vi "is_inside.vi"(8 "error in (no error)":errorcluster, 10 "SpaceVector.lvclass":refnum<class "SpaceVector.lvclass">, 11 "ROI in":refnum<class "RoiEllipsoid.lvclass">=refnum) -> (0 "error out":errorcluster, 2 "is inside?":bool, 3 "ROI out":refnum<class "RoiEllipsoid.lvclass">)   [LabVIEW 2010, in "RoiEllipsoid.lvclass"]
uses:
  RoiEllipsoid.lvclass
  common/classes/SpaceVector/SpaceVector/SpaceVector.lvclass
  RoiGeneric/RoiGeneric.lvclass
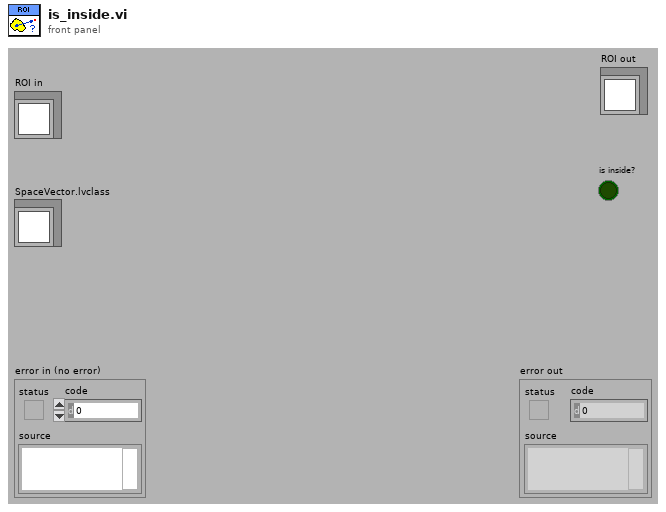
[diagram p1: front panel]
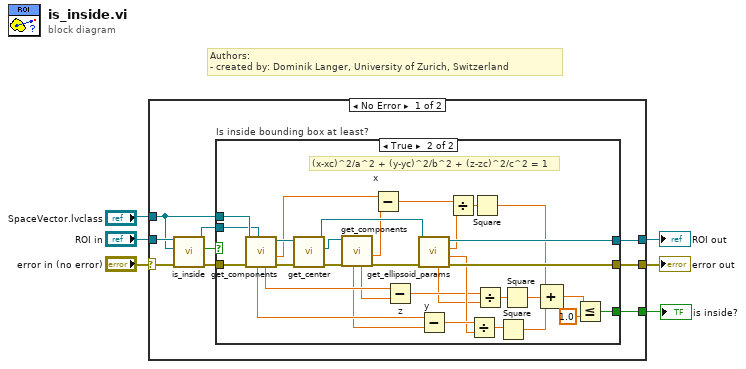
[diagram p0: block diagram]
diagram:
  # "Authors: \n- created by: Dominik Langer, University of Zurich, Switzerland"
  n1 = case shown="No Error" "error in (no error)" {
    selector: "error in (no error)" -> [w15 w50]
    tunnel: "ROI in" -> [w14 w49]
    tunnel: "SpaceVector.lvclass" -> [w13 _]
    tunnel: [w10 w50] -> w3
    tunnel: [w8 w49] -> w2
    tunnel: [w7 _] -> w1
    frame No Error {
      n2 = call-parent "is_inside.vi"("error in (no error)"=w15, "SpaceVector.lvclass"=w13, "ROI in"=w14) -> ("error out"=w12:errorcluster, "is inside?"=w11:bool, "ROI out"=w9:refnum<class "RoiEllipsoid.lvclass">)  [unwired: 6 in]
      n3 = case "Is inside bounding box at least?" shown="True" w11 {
        tunnel: w13 -> [_ w48]
        tunnel: w12 -> [w17 w47]
        tunnel: [w17 w46] -> w10
        tunnel: w9 -> [w16 w44]
        tunnel: [w16 w45] -> w8
        tunnel: [_ w18] -> w7
        frame False {
        }
        frame True {
          # "(x-xc)^2/a^2 + (y-yc)^2/b^2 + (z-zc)^2/c^2 = 1"
          n4 = call "get_components.vi"("error in (no error)"=w47, "SpaceVector in"=w48) -> ("error out"=w43:errorcluster, "x"=w38:dbl[unit], "z"=w36:dbl[unit], "y"=w34:dbl[unit])  [unwired: 4 in, 2 out]
          n5 = call-dynamic "get_center.vi"("error in (no error)"=w43, "RoiGeneric in"=w44) -> ("error out"=w40:errorcluster, "center"=w41:refnum<class "SpaceVector.lvclass">, "RoiGeneric out"=w42:refnum<class "RoiEllipsoid.lvclass">)  [unwired: 7 in]
          n6 = call "get_components.vi"("error in (no error)"=w40, "SpaceVector in"=w41) -> ("error out"=w39:errorcluster, "x"=w37:dbl[unit], "z"=w35:dbl[unit], "y"=w33:dbl[unit])  [unwired: 4 in, 2 out]
          n7 = Subtract "x"(x=w38, y=w37) -> (x-y=w32:dbl[unit])
          n8 = Subtract "z"(x=w36, y=w35) -> (x-y=w27:dbl[unit])
          n9 = call-dynamic "get_ellipsoid_params.vi"("error in (no error)"=w39, "RoiEllipsoid in"=w42) -> ("error out"=w46:errorcluster, "b"=w28:dbl[unit], "a"=w31:dbl[unit], "RoiEllipsoid out"=w45:refnum<class "RoiEllipsoid.lvclass">, "c"=w26:dbl[unit])  [unwired: 5 in]
          n10 = Subtract "y"(x=w34, y=w33) -> (x-y=w29:dbl[unit])
          n11 = Divide(x=w32, y=w31) -> (x/y=w30:dbl)
          n12 = Divide(x=w29, y=w28) -> (x/y=w24:dbl)
          n13 = Square(x=w30) -> (x^2=w23:dbl)
          n14 = Divide(x=w27, y=w26) -> (x/y=w25:dbl)
          n15 = Square(x=w24) -> (x^2=w21:dbl)
          n16 = Square(x=w25) -> (x^2=w22:dbl)
          n17 = Compound Arithmetic op=ADD(w23, w22, w21) -> (w20:dbl)
          n18 = Less Or Equal?(x=w20, y=1.0) -> (x <= y?=w18:bool)
        }
      }
    }
    frame Error {
    }
  }
  "error out" <- w3
  "ROI out" <- w2
  "is inside?" <- w1
